vi "DAQmx_Pulse_GenerateAccordingInput.vi"() -> ()   [LabVIEW 2025]
doc: "This example demonstrates how to generate a single pulse using a counter output. \n\nThe single pulse may be triggered once or repeatedly from an external source."
uses:
  <vilib>/Utility/error.llb/DialogType.ctl
  <vilib>/DAQmx/create/channels.llb/DAQmx Create Channel (CO-Pulse Generation-Time).vi
  <vilib>/DAQmx/configure/trigger.llb/DAQmx Start Trigger (Digital Edge).vi
  <resource>/objmgr/daqmx.rc
panel:
  in  "Digital Trigger Source":tag="/Dev1/PFI0"
  in  "Pulse Duration":dbl=0.00025 format="%.6f"
  in  "Output Terminal":tag="/Dev1/PFI12"
  in  "Stop":bool
  in  "Counter":tag="Dev1/ctr0"
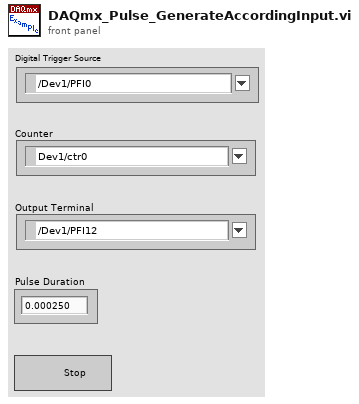
[diagram p1: front panel]
types:
  T1 = typedef "DialogType.ctl" = u16
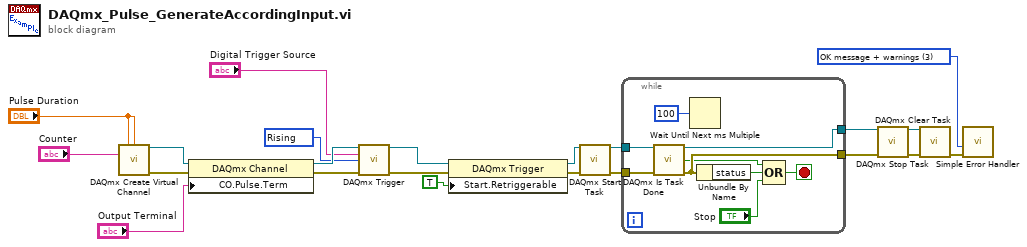
[diagram p0: block diagram]
diagram:
  w3 = 10280 items=["Rising"=10280, "Falling"=10171] ("Edge")
  w8 = T1 3 items=["no dialog", "OK message", "continue or stop message", "OK message + warnings", "continue/stop + warnings"] ("type of dialog (OK msg:1)")
  n1 = call-poly <vilib>:"DAQmx Create Virtual Channel.vi"("high time"="Pulse Duration", "low time"="Pulse Duration", "counter"="Counter") -> ("task out"=w18:refnum<k21>, "error out"=w17:errorcluster)  [unwired: 11 in]
  n2 = property class="DAQmx Channel"(reference=w18, error in=w17, "CO.Pulse.Term"="Output Terminal") -> (reference out=w14:refnum<k21>, error out=w15:errorcluster)
  n3 = call-poly <vilib>:"DAQmx Trigger.vi"("task/channels in"=w14, "source"="Digital Trigger Source", "edge"=w3, "error in"=w15) -> ("task out"=w6:refnum<k21>, "error out"=w5:errorcluster)  [unwired: 10 in]
  n4 = property class="DAQmx Trigger"(reference=w6, error in=w5, "Start.Retriggerable"=TRUE ("Retriggerable")) -> (reference out=w2:refnum<k21>, error out=w1:errorcluster)
  n5 = call <vilib>:"DAQmx Start Task.vi"("task/channels in"=w2, "error in"=w1) -> ("task out"=w22:refnum<k21>, "error out"=w21:errorcluster)  [unwired: 12 in]
  n6 = while {
    tunnel: w22 -> [w31]
    tunnel: w21 -> [w30]
    tunnel: [w27] -> w11
    tunnel: [w28] -> w12
    stop <- w29 stop-if-true
    n7 = call <vilib>:"DAQmx Is Task Done.vi"("task/channels in"=w31, "error in"=w30) -> ("task out"=w28:refnum<k21>, "task done?"=w23:bool, "error out"=w27:errorcluster)  [unwired: 11 in]
    n8 = Wait Until Next ms Multiple(millisecond multiple=u32 100) -> ()  [unwired: 1 out]
    n9 = Unbundle By Name(w27) -> ("status"=w26:bool)
    n10 = Compound Arithmetic op=OR(w23, w26, "Stop") -> (w29:bool)
  }
  n11 = call <vilib>:"DAQmx Stop Task.vi"("task/channels in"=w12, "error in"=w11) -> ("task out"=w10:refnum<k21>, "error out"=w9:errorcluster)  [unwired: 12 in]
  n12 = call <vilib>:"DAQmx Clear Task.vi"("task in"=w10, "error in"=w9) -> ("error out"=w20:errorcluster)  [unwired: 13 in]
  n13 = call <vilib>:"Simple Error Handler.vi"("type of dialog (OK msg:1)"=w8, "error in (no error)"=w20) -> ()  [unwired: 3 in, 5 out]
